vi "PIV_Init.vi"() -> (0 "error out":errorcluster)   [LabVIEW 2025]
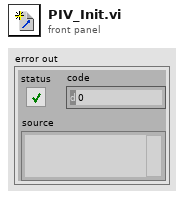
[diagram p1: front panel]
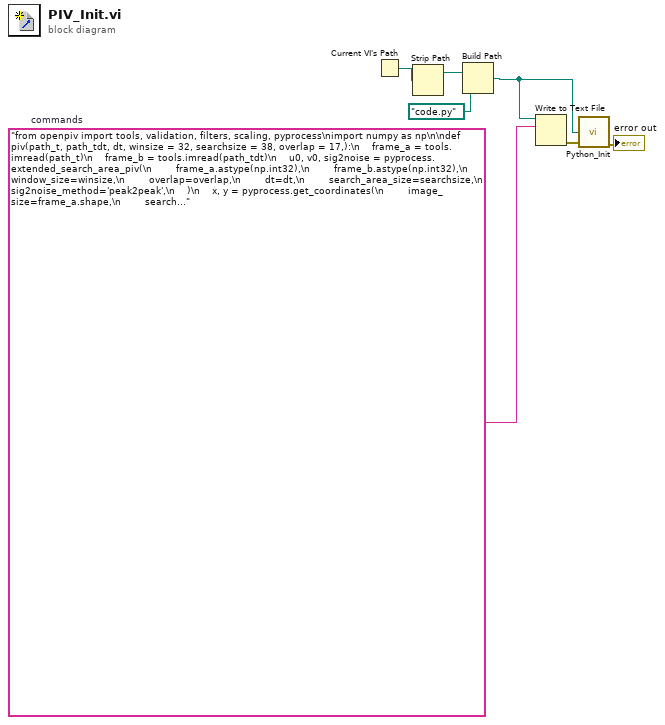
[diagram p0: block diagram]
diagram:
  w5 = "from openpiv import tools, validation, filters, scaling, pyprocess\nimport numpy as np\n\ndef piv(path_t, path_tdt, dt, winsize = 32, searchsize = 38, overlap = 17,):\n    frame_a = tools.imread(path_t)\n    frame_b = tools.imread(path_tdt)\n    u0, v0, sig2noise = pyprocess.extended_search_area_piv(\n        frame_a.astype(np.int32),\n        frame_b.astype(np.int32),\n        window_size=winsize,\n        overlap=overlap,\n        dt=dt,\n        search_area_size=searchsize,\n        sig2noise_method='peak2peak',\n    )\n    x, y = pyprocess.get_coordinates(\n        image_size=frame_a.shape,\n        search_area_size=searchsize,\n        overlap=overlap,\n    )\n    #mask = validation.sig2noise_val(sig2noise, 1.05)\n    return (x.tolist(), y.tolist(), u0.tolist(), v0.tolist(), sig2noise.tolist())\n\ndef interpolate(u0, v0, sig2noise, method, max_iter, kernel_size):\n    mask = validation.sig2noise_val(sig2noise, 1.05)\n    u2, v2 = filters.replace_outliers(\n        u0, v0,\n        mask,\n        method='localmean',\n        max_iter=3,\n        kernel_size=3,\n    )\n    return (u2.tolist(), v2.tolist())\n\n# convert x,y to mm\n# convert u,v to mm/sec\n\ndef scale(scaling_factor, dt, x, y, u2 ,v2):\n    x, y, u3, v3 = scaling.uniform(\n        x, y, u2, v2, scaling_factor,  #  in pixels/millimeter\n    )\n    # 0,0 shall be bottom left, positive rotation rate is counterclockwise\n    x, y, u3, v3 = tools.transform_coordinates(x, y, u3, v3)\n    return (x, y, u3, v3)\n"  # commands
  n1 = Current VI's Path() -> (path=w3:path)
  n2 = Strip Path(path=w3) -> (stripped path=w4:path)  [unwired: 1 out]
  n3 = Build Path(base path=w4, name or relative path=path "code.py" ("file (use dialog)")) -> (appended path=w1:path)
  n4 = Write to Text File(file (use dialog)=w1, text=w5) -> (error out=w6:errorcluster)  [unwired: 2 in, 2 out]
  n5 = call "Python_Init.vi"("code in"=w1, "error in (no error)"=w6) -> ("error out"=→"error out":errorcluster)  [unwired: 2 in, 2 out]
